vi "View.vi"(8 "error in (no error)":errorcluster, 11 "Device Under Test In":refnum<class "Device Under Test.lvclass">) -> (0 "error out":errorcluster)   [LabVIEW 2020, in "Device Under Test.lvclass"]
doc: "This VI implements the main UI of the process. A reference to this VI should be set using the Set View VI Reference.vi method when the VI is started."
uses:
  Device Under Test.lvclass
  Device Under Test.lvclass/Device Under Test.ctl
  <vilib>/Astemes/Triarc Framework/View/View.lvclass
  <vilib>/Astemes/Triarc Framework/Process/Process.lvclass
  C:/Program Files (x86)/National Instruments/LabVIEW 2020/vi.lib/Asteme/Triarc Framework/View/View.lvclass
  C:/Program Files (x86)/National Instruments/LabVIEW 2020/vi.lib/Asteme/Triarc Framework/Process/Process.lvclass
  C:/Program Files (x86)/National Instruments/LabVIEW 2020/vi.lib/Asteme/Triarc Framework/Base/Base.lvclass
  C:/Program Files (x86)/National Instruments/LabVIEW 2020/vi.lib/Asteme/Triarc Framework/Error Handler Interface/Error Handler Interface.lvclass
  C:/Program Files (x86)/National Instruments/LabVIEW 2020/vi.lib/Asteme/Triarc Framework/Logging/Logging.lvclass
  C:/Users/anton/Documents/GitHub/Triarc-Examples/Thermal Chamber/Device Under Test/Device Under Test.lvclass
panel:
  out "Status":string
  in  "Self Test":bool
  in  "Power Off":bool
  in  "Power On":bool
  out "Self Test Result":bool
  out "Power  State":bool
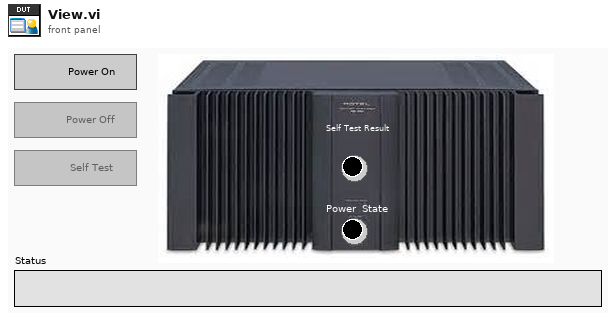
[diagram p1: front panel]
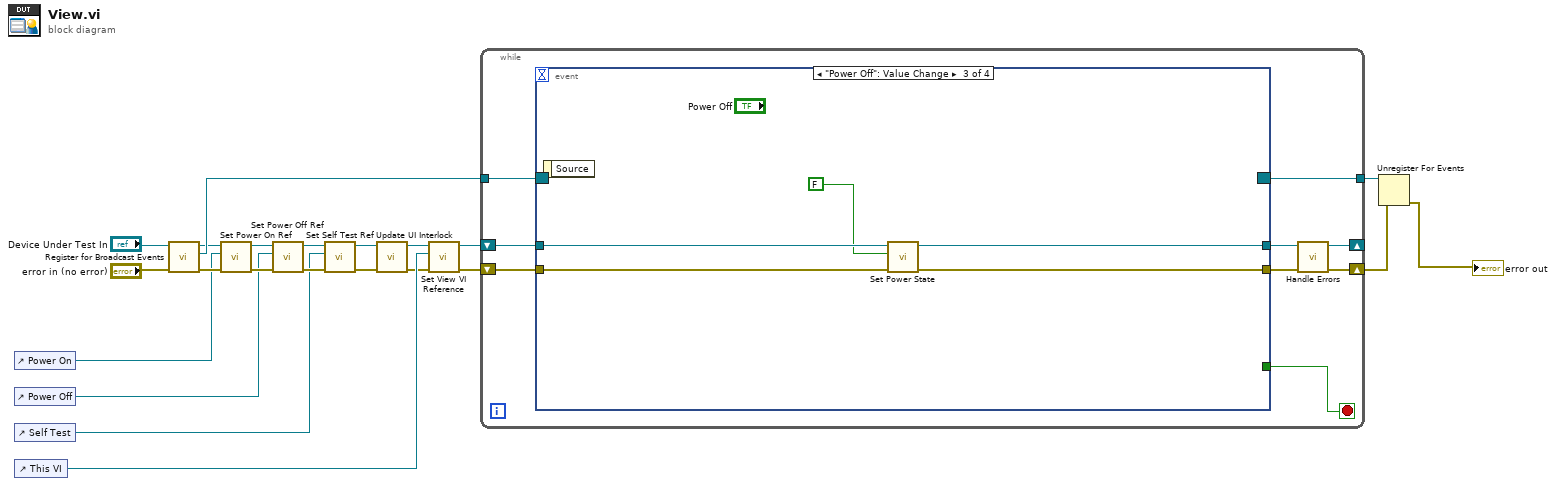
[diagram p0: block diagram]
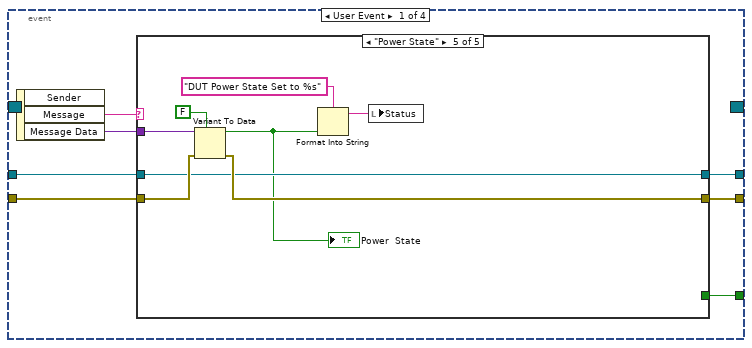
[diagram p2: hidden frame]
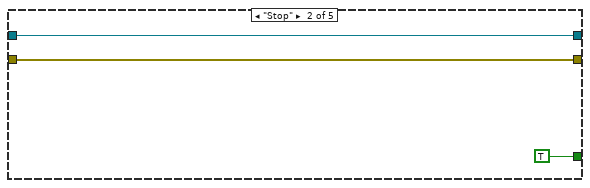
[diagram p4: hidden frame]
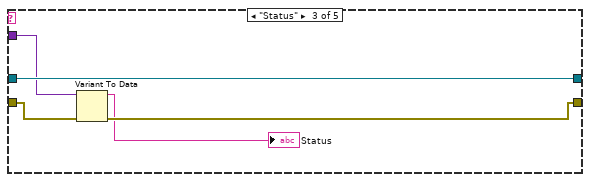
[diagram p5: hidden frame]
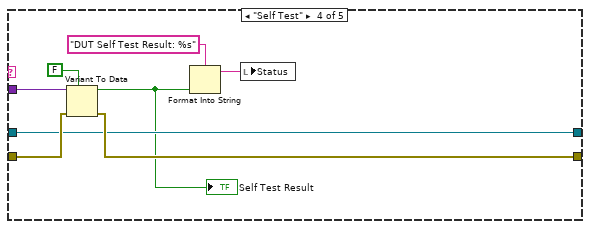
[diagram p6: hidden frame]
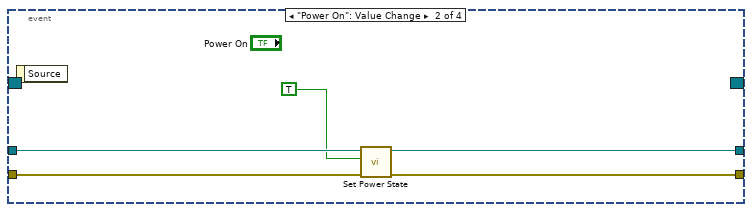
[diagram p7: hidden frame]
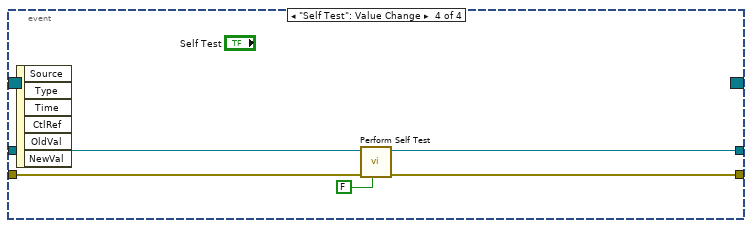
[diagram p8: hidden frame]
diagram:
  n1 = control-ref of="Power On"() -> (w6:refnum<vi>)
  n2 = control-ref of="Power Off"() -> (w5:refnum<vi>)
  n3 = control-ref of="Self Test"() -> (w4:refnum<vi>)
  n4 = control-ref of="This VI"() -> (w14:refnum<vi>)
  n5 = call <vilib>:"Register for Broadcast Events.vi"("error in (no error)"="error in (no error)", "Process In"="Device Under Test In") -> ("error out"=w12:errorcluster, "Event Registration Refnum Out"=w19:refnum<event-registration>, "Process Out"=w13:refnum<class "Device Under Test.lvclass">)  [unwired: 7 in]
  n6 = call "Set Power On Ref.vi"("error in (no error)"=w12, "Self Test"=w6, "Device Under Test In"=w13) -> ("error out"=w10:errorcluster, "Device Under Test Out"=w11:refnum<class "Device Under Test.lvclass">)  [unwired: 7 in]
  n7 = call "Set Power Off Ref.vi"("error in (no error)"=w10, "Self Test"=w5, "Device Under Test In"=w11) -> ("error out"=w8:errorcluster, "Device Under Test Out"=w9:refnum<class "Device Under Test.lvclass">)  [unwired: 7 in]
  n8 = call "Set Self Test Ref.vi"("error in (no error)"=w8, "Self Test"=w4, "Device Under Test In"=w9) -> ("error out"=w7:errorcluster, "Device Under Test Out"=w2:refnum<class "Device Under Test.lvclass">)  [unwired: 7 in]
  n9 = call "Update UI Interlock.vi"("error in (no error)"=w7, "Device Under Test In"=w2) -> ("error out"=w3:errorcluster, "Device Under Test Out"=w1:refnum<class "Device Under Test.lvclass">)  [unwired: 8 in]
  n10 = call <vilib>:"Set View VI Reference.vi"("error in (no error)"=w3, "View VI Reference"=w14, "View In"=w1) -> ("error out"=w18:errorcluster, "View Out"=w17:refnum<class "Device Under Test.lvclass">)  [unwired: 7 in]
  n11 = while {
    shift-right: [w25] -> _
    shift-left: w17 -> [w31]
    shift-right: [w23] -> w16
    shift-left: w18 -> [w29]
    tunnel: w19 -> [w28]
    tunnel: [w27] -> w15
    stop <- w26 stop-if-true
    n12 = event shown="[2] \"Power Off\": Value Change" {
      selector: w28 -> [_ _ _ _]
      dyn-events: [_ _ _ _] -> w27
      timeout: _ -> [_ _ _ _]
      tunnel: w31 -> [w38 w67 w72 w77]
      tunnel: [w37 w66 w71 w76] -> w30
      tunnel: w29 -> [w35 w69 w74 w79]
      tunnel: [w36 w68 w73 w78] -> w24
      tunnel: [w33 _ _ _] -> w26
      event User Event {
        n13 = event-data() -> ("Message"=w34:string, "Message Data"=w32:variant)  [unwired: 1 in, 1 out]
        n14 = case shown="\"Power State\"" w34 {
          tunnel: w38 -> [w40 w43 w48 w50 w58]
          tunnel: [w40 w43 w48 w50 w58] -> w37
          tunnel: [w39 w42 w46 w51 w59] -> w36
          tunnel: w35 -> [w39 w42 w47 w54 w62]
          tunnel: [_ TRUE _ _ _] -> w33
          tunnel: w32 -> [_ _ w45 w56 w64]
          frame Default {
          }
          frame "Stop" {
          }
          frame "Status" {
            n15 = Variant To Data(error in=w47, Variant=w45) -> (data=→"Status":string, error out=w46:errorcluster)  [unwired: 1 in]
          }
          frame "Self Test" {
            n16 = Variant To Data(error in=w54, type=FALSE, Variant=w56) -> (data=w49:bool, error out=w51:errorcluster)
            "Self Test Result" <- w49
            n17 = Format Into String(format string="DUT Self Test Result: %s", w49) -> (resulting string=w52:string)  [unwired: 2 in, 1 out]
            n18 = local write "Status"(w52) -> ()
          }
          frame "Power State" {
            n19 = Variant To Data(error in=w62, type=FALSE, Variant=w64) -> (data=w57:bool, error out=w59:errorcluster)
            "Power  State" <- w57
            n20 = Format Into String(format string="DUT Power State Set to %s", w57) -> (resulting string=w60:string)  [unwired: 2 in, 1 out]
            n21 = local write "Status"(w60) -> ()
          }
        }
      }
      event "Power On": Value Change {
        n22 = event-data() -> ()  [unwired: 1 in, 1 out]
        n23 = call "Set Power State.vi"("error in (no error)"=w69, "Power State"=TRUE, "Device Under Test In"=w67) -> ("error out"=w68:errorcluster, "Device Under Test Out"=w66:refnum<class "Device Under Test.lvclass">)  [unwired: 7 in]
      }
      event "Power Off": Value Change {
        n24 = event-data() -> ()  [unwired: 1 in, 1 out]
        n25 = call "Set Power State.vi"("error in (no error)"=w74, "Power State"=FALSE, "Device Under Test In"=w72) -> ("error out"=w73:errorcluster, "Device Under Test Out"=w71:refnum<class "Device Under Test.lvclass">)  [unwired: 7 in]
      }
      event "Self Test": Value Change {
        n26 = event-data() -> ()  [unwired: 1 in, 6 out]
        n27 = call "Perform Self Test.vi"("Wait for Reply?"=FALSE, "error in (no error)"=w79, "Device Under Test In"=w77) -> ("error out"=w78:errorcluster, "Device Under Test Out"=w76:refnum<class "Device Under Test.lvclass">)  [unwired: 5 in, 2 out]
      }
    }
    n28 = call-dynamic "Handle Errors.vi"("error in (no error)"=w24, "Process In"=w30) -> ("error out"=w23:errorcluster, "Process Out"=w25:refnum<class "Device Under Test.lvclass">)  [unwired: 8 in]
  }
  n29 = Unregister For Events(event registration refnum=w15, error in=w16) -> (error out=→"error out":errorcluster)
